vi "SSH Unix Session FGV.vi"(9 "info in":T1={"PID"=-1, "Read FD"=-1, "Write FD"=-1, "Error FD"=-1}, 10 "Session In":i32=1, 11 "Operation":T2) -> (2 "info in":T1={"PID"=-1, "Read FD"=-1, "Write FD"=-1, "Error FD"=-1}, 3 "Session Out":i32=1)   [LabVIEW 2020, in "LMH-LINX.lvlib"]
uses:
  LMH-LINX.lvlib
  SSH Unix Session Op.ctl
  SSH Unix Session Info.ctl
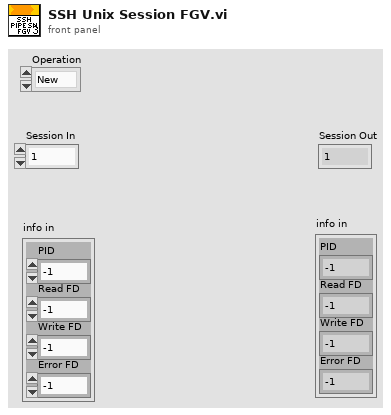
[diagram p1: front panel]
types:
  T1 = typedef "LMH-LINX.lvlib/SSH Unix Session Info.ctl" = cluster{"PID":i32, "Read FD":i32, "Write FD":i32, "Error FD":i32}
  T2 = typedef "LMH-LINX.lvlib/SSH Unix Session Op.ctl" = enum16{"New", "Get", "Delete"}
  T3 = cluster{"PID":i32, "Read FD":i32, "Write FD":i32, "Error FD":i32}
  T4 = map{i32, cluster{"PID":i32, "Read FD":i32, "Write FD":i32, "Error FD":i32}}
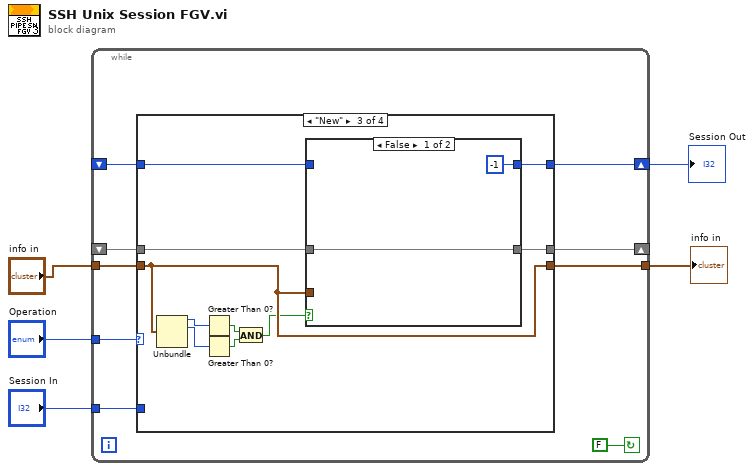
[diagram p0: block diagram]
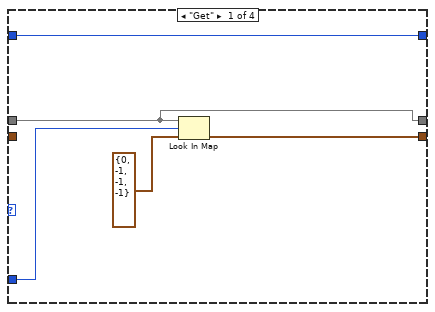
[diagram p2: hidden frame]
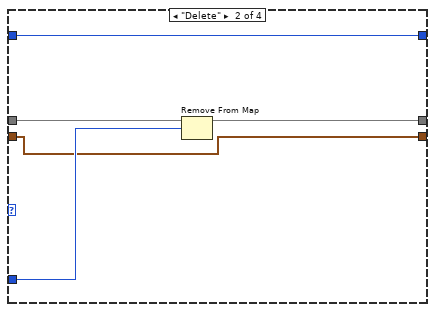
[diagram p3: hidden frame]
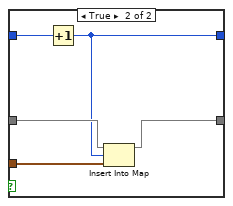
[diagram p4: hidden frame]
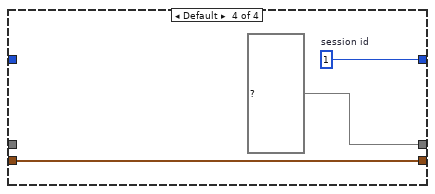
[diagram p5: hidden frame]
diagram:
  n1 = while {
    shift-right: [w12] -> _
    shift-left: _ -> [w14]
    tunnel: "Operation" -> [w13]
    tunnel: "Session In" -> [w11]
    shift-right: [w10] -> w2
    shift-left: _ -> [w9]
    tunnel: [w7] -> w3
    tunnel: "info in" -> [w6]
    stop <- FALSE continue-if-true
    n2 = case shown="\"New\"" w13 {
      tunnel: w14 -> [w19 w24 w34 _]
      tunnel: [w19 w23 w33 T4 {} ("map in")] -> w12
      tunnel: w11 -> [w17 w22 _ _]
      tunnel: [w18 w21 w31 w43] -> w10
      tunnel: w9 -> [w18 w21 w32 _]
      tunnel: [w15 w20 w30 w42] -> w7
      tunnel: w6 -> [_ w20 w30 w42]
      frame "Get" {
        n3 = Look In Map(map=w19, key=w17, default value=T3 {"PID"=0, "Read FD"=-1, "Write FD"=-1, "Error FD"=-1}) -> (value=w15:T3)  [unwired: 1 out]
      }
      frame "Delete" {
        n4 = Remove From Map(10:w22, 11:w24) -> (3:w23:T4)  [unwired: 2 out]
      }
      frame "New" {
        n5 = Unbundle(w30) -> ("PID"=w29:i32, "Read FD"=w28:i32)  [unwired: 2 out]
        n6 = Greater Than 0?(x=w29) -> (x > 0?=w27:bool)
        n7 = Greater Than 0?(x=w28) -> (x > 0?=w26:bool)
        n8 = And(x=w27, y=w26) -> (x .and. y?=w25:bool)
        n9 = case shown="False" w25 {
          tunnel: w34 -> [w36 w41]
          tunnel: [w36 w40] -> w33
          tunnel: w32 -> [_ w39]
          tunnel: [-1 w38] -> w31
          tunnel: w30 -> [_ w37]
          frame False {
          }
          frame True {
            n10 = Increment(x=w39) -> (x+1=w38:i32)
            n11 = Insert Into Map(map in=w41, key=w38, value=w37) -> (map out=w40:T4)  [unwired: 2 out]
          }
        }
      }
      frame Default {
        w43 = 1  # session id
      }
    }
  }
  "info in" <- w3
  "Session Out" <- w2
